vi "Enum To String Scripter.vi"(8 "Error In":errorcluster, 11 "Enum Path":path=path "C:/Users/samkristoff/Desktop/output.ctl") -> (0 "Error Out":errorcluster)   [LabVIEW 2014, in "LMH-Toolbox.lvlib" / "LMH-Scripting.lvlib"]
doc: "Script a VI that returns the string name of the specified enum index without using property nodes. This is particularly useful when deploying to RT targets where the front panel is stripped."
uses:
  <vilib>/MakerHub/Toolbox/Private/Scripting/LMH-Scripting.lvlib
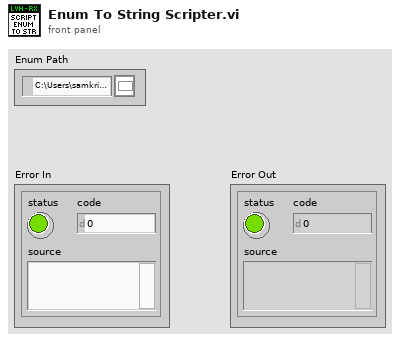
[diagram p1: front panel]
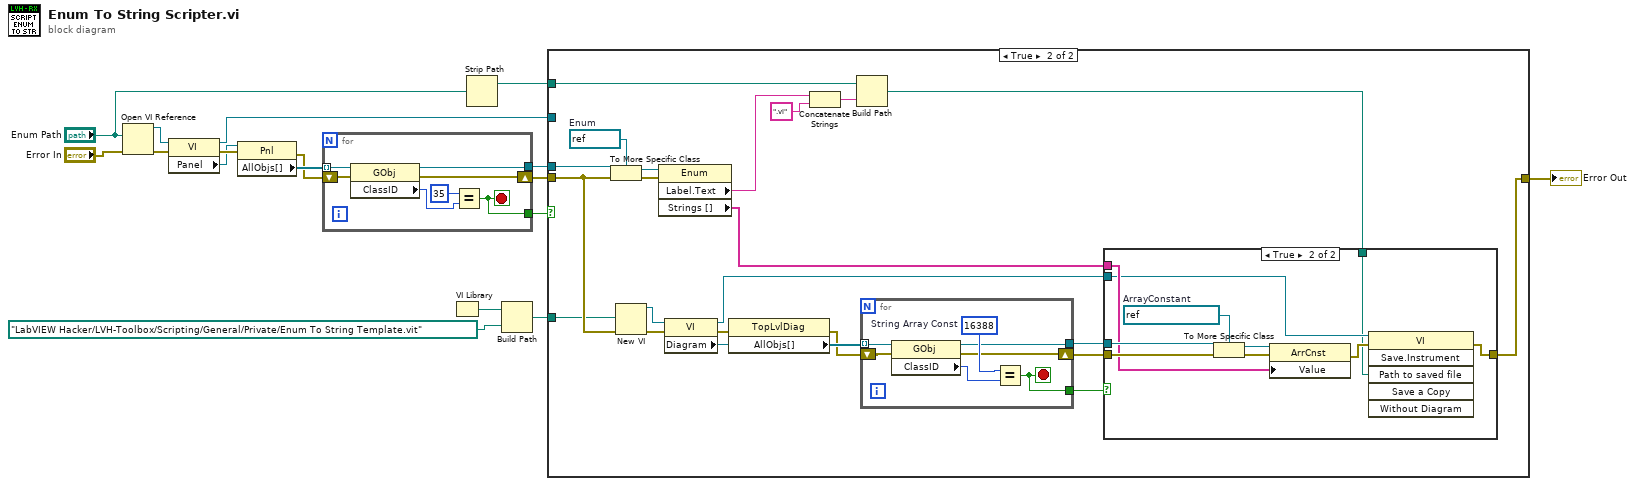
[diagram p0: block diagram]
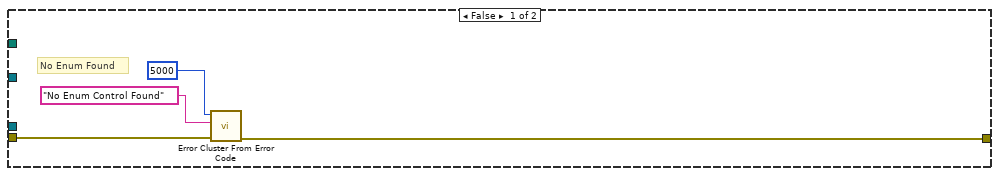
[diagram p2: hidden frame]
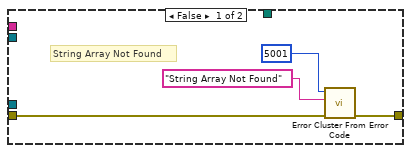
[diagram p3: hidden frame]
diagram:
  n1 = Open VI Reference(vi path="Enum Path", error in (no error)="Error In") -> (vi reference=w16:refnum<vi>, error out=w15:errorcluster)  [unwired: 4 in]
  n2 = property class="VI"(reference=w16, error in=w15) -> (reference out=w5:refnum<vi>, error out=w17:errorcluster, "Panel"=w14:refnum<vi>)
  n3 = property class="Pnl"(reference=w14, error in=w17) -> (error out=w12:errorcluster, "AllObjs[]"=w13:refnum<vi>[])  [unwired: 1 out]
  n4 = for {
    tunnel: w13 -> [w24] mode=indexing
    shift-right: [w20] -> w9
    shift-left: w12 -> [w21]
    tunnel: [w19] -> w10
    tunnel: [w18] -> w11
    stop <- w19 stop-if-true
    n5 = property class="GObj"(reference=w24, error in=w21) -> (reference out=w18:refnum<vi>, error out=w20:errorcluster, "ClassID"=w23:u32)
    n6 = Equal?(x=u32 35, y=w23) -> (x = y?=w19:bool)
  }
  n7 = VI Library() -> (path=w8:path)
  n8 = Strip Path(path="Enum Path") -> (stripped path=w2:path)  [unwired: 1 out]
  n9 = Build Path(base path=w8, name or relative path=path "LabVIEW Hacker/LVH-Toolbox/Scripting/General/Private/Enum To String Template.vit" ("path")) -> (appended path=w6:path)
  n10 = case shown="True" w10 {
    tunnel: w11 -> [_ w51]
    tunnel: w9 -> [w28 w47]
    tunnel: [w25 w36] -> w4
    tunnel: w6 -> [_ w46]
    tunnel: w5 -> [_ _]
    tunnel: w2 -> [_ w33]
    frame False {
      # "No Enum Found"
      n11 = call <vilib>:"Error Cluster From Error Code.vi"("error in (no error)"=w28, "error message (\"\")"="No Enum Control Found" ("error message (\"\")"), "error code (0)"=5000) -> ("error out"=w25:errorcluster)  [unwired: 6 in]
    }
    frame True {
      w50 = refnum<vi> refnum  # Enum
      n12 = To More Specific Class(target class=w50, reference=w51, error in=w47) -> (specific class reference=w49:refnum<vi>, error out=w48:errorcluster)
      n13 = New VI(8:w47, 10:w46) -> (0:w43:errorcluster, 3:w42:refnum<vi>)  [unwired: 5 in]
      n14 = property class="Enum"(reference=w49, error in=w48) -> ("Label.Text"=w31:string, "Strings []"=w34:string[])  [unwired: 2 out]
      n15 = property class="VI"(reference=w42, error in=w43) -> (reference out=w37:refnum<vi>, error out=w44:errorcluster, "Diagram"=w45:refnum<vi>)
      n16 = property class="TopLvlDiag"(reference=w45, error in=w44) -> (error out=w40:errorcluster, "AllObjs[]"=w41:refnum<vi>[])  [unwired: 1 out]
      n17 = Concatenate Strings(w31, ".vi" ("string")) -> (w32:string)
      n18 = Build Path(base path=w33, name or relative path=w32) -> (appended path=w29:path)
      n19 = for {
        tunnel: w41 -> [w67] mode=indexing
        shift-right: [w70] -> w39
        shift-left: w40 -> [w71]
        tunnel: [w69] -> w35
        tunnel: [w68] -> w38
        tunnel: [w67] -> _ mode=indexing
        stop <- w69 stop-if-true
        w72 = u32 16388  # String Array Const
        n20 = property class="GObj"(reference=w67, error in=w71) -> (reference out=w68:refnum<vi>, error out=w70:errorcluster, "ClassID"=w66:u32)
        n21 = Equal?(x=w72, y=w66) -> (x = y?=w69:bool)
      }
      n22 = case shown="True" w35 {
        tunnel: w39 -> [w52 w65]
        tunnel: w38 -> [_ w64]
        tunnel: w34 -> [_ w60]
        tunnel: w37 -> [_ w59]
        tunnel: [w53 w57] -> w36
        tunnel: w29 -> [_ w56]
        frame False {
          # "String Array Not Found"
          n23 = call <vilib>:"Error Cluster From Error Code.vi"("error in (no error)"=w52, "error message (\"\")"="String Array Not Found" ("error message (\"\")"), "error code (0)"=5001) -> ("error out"=w53:errorcluster)  [unwired: 6 in]
        }
        frame True {
          w63 = refnum<vi> refnum  # ArrayConstant
          n24 = To More Specific Class(target class=w63, reference=w64, error in=w65) -> (specific class reference=w62:refnum<vi>, error out=w61:errorcluster)
          n25 = property class="ArrCnst"(reference=w62, error in=w61, "Value"=w60) -> (error out=w58:errorcluster)  [unwired: 1 out]
          n26 = invoke class="VI" method="Save.Instrument"(reference=w59, error in=w58, "Path to saved file"=w56) -> (error out=w57:errorcluster)  [unwired: 3 in, 5 out]
        }
      }
    }
  }
  "Error Out" <- w4
